vi "Qs_adapt-qd_sd-de-delai@20.vi"(5 "error in (no error)":errorcluster caption="entrée d'erreur (pas d'erreur)", 6 "Sigma":dbl, 7 "Moyenne":dbl, 8 "Durée":dbl, 9 "Délai d":dbl) -> (0 "Sigma d":dbl, 2 "Qd":dbl, 4 "error out":errorcluster caption="sortie d'erreur")   [LabVIEW 2010, in "lv_07.lvlib"]
doc: "Durée est la période pour laquelle les caractéristiques de consommation mesurées par l'entreprise (moyenne et écart-type) sont données. Le délai d est le délai imposé par les conditions d'approvisionnement (fournisseur).\nQd et Sigma d sont les caractéristiques appliquées au modèle statistique approprié (Poisson si Qd faible, ou Loi Normale)"
uses:
  lv_07.lvlib
  lv_02/lv_02.lvlib
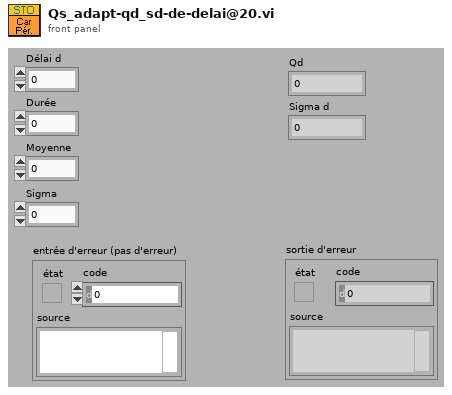
[diagram p1: front panel]
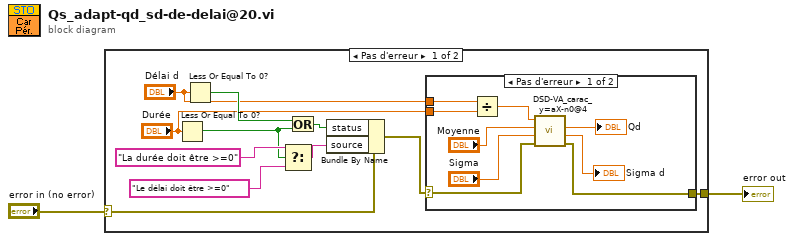
[diagram p0: block diagram]
diagram:
  n1 = case shown="Pas d'erreur" "error in (no error)" {
    selector: "error in (no error)" -> [w13 w24]
    tunnel: [w3 w24] -> w1
    frame No Error {
      n2 = Less Or Equal To 0?(x="Durée") -> (x <= 0?=w8:bool)
      n3 = Less Or Equal To 0?(x="Délai d") -> (x <= 0?=w9:bool)
      n4 = Select(t="La durée doit être >=0" ("source"), s=w8, f="Le délai doit être >=0" ("source")) -> (s? t:f=w10:string)
      n5 = Or(x=w9, y=w8) -> (x .or. y?=w7:bool)
      n6 = Bundle By Name(cluster=w13, "status"=w7, "source"=w10) -> (w4:errorcluster)
      n7 = case shown="Pas d'erreur" w4 {
        selector: w4 -> [w17 w23]
        tunnel: "Délai d" -> [w22 _]
        tunnel: "Durée" -> [w21 _]
        tunnel: [w16 w23] -> w3
        frame No Error {
          n8 = Divide(x=w22, y=w21) -> (x/y=w20:dbl)
          n9 = call "DSD-VA_carac_y=aX-n0@4.vi"("error in (no error)"=w17, "S_X"="Sigma", "E(X)"="Moyenne", "a"=w20) -> ("error out"=w16:errorcluster, "S_aX"=→"Sigma d":dbl, "E(a.X)"=→"Qd":dbl)  [unwired: 5 in]
        }
        frame Error {
        }
      }
    }
    frame Error {
    }
  }
  "error out" <- w1
